vi "Gaussian_Values_Create.vi"(1 "offset":dbl, 2 "X-Axis":dbl[](array[numeric]), 5 "amplitude":dbl, 7 "center":dbl format="%.1f", 9 "sigma":dbl format="%.1f") -> (6 "Gaussian (Y)":dbl[](array[numeric]))   [LabVIEW 2018]
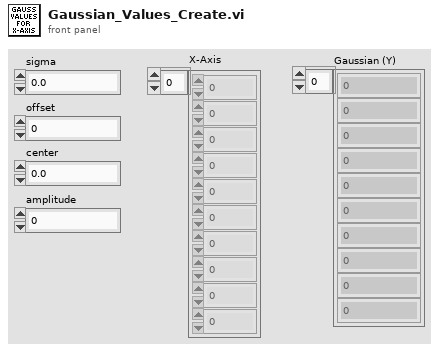
[diagram p1: front panel]
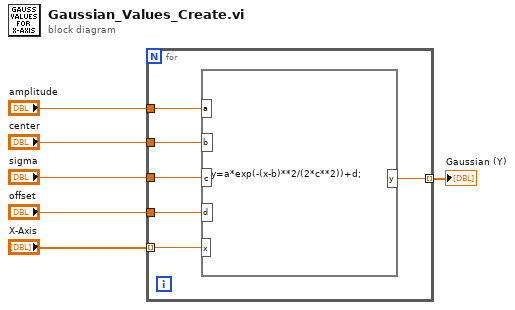
[diagram p0: block diagram]
diagram:
  n1 = for {
    tunnel: "amplitude" -> [w12]
    tunnel: "center" -> [w11]
    tunnel: "sigma" -> [w10]
    tunnel: "offset" -> [w9]
    tunnel: "X-Axis" -> [w8] mode=indexing
    tunnel: [w7] -> w1 mode=indexing
    n2 = formula code="y=a*exp(-(x-b)**2/(2*c**2))+d;"("a"=w12, "b"=w11, "c"=w10, "d"=w9, "x"=w8) -> ("y"=w7:dbl)
  }
  "Gaussian (Y)" <- w1
